vi "Initialize Components.vi"(7 "Components":refnum<class "Component.lvclass">[](array[class]), 8 "error in (no error)":errorcluster, 10 "Plugin Configuration":refnum<class "Plugin Configuration.lvclass">, 11 "Plugin Thread in":refnum<class "Plugin Thread.lvclass">) -> (0 "error out":errorcluster, 3 "Plugin Thread out":refnum<class "Plugin Thread.lvclass">)   [LabVIEW 2019, in "DSF Core.lvlib" / "Plugin Thread.lvclass"]
uses:
  Plugin Thread.lvclass
  Component/Component.lvclass
  Configuration/Core/Plugin/Plugin Configuration.lvclass
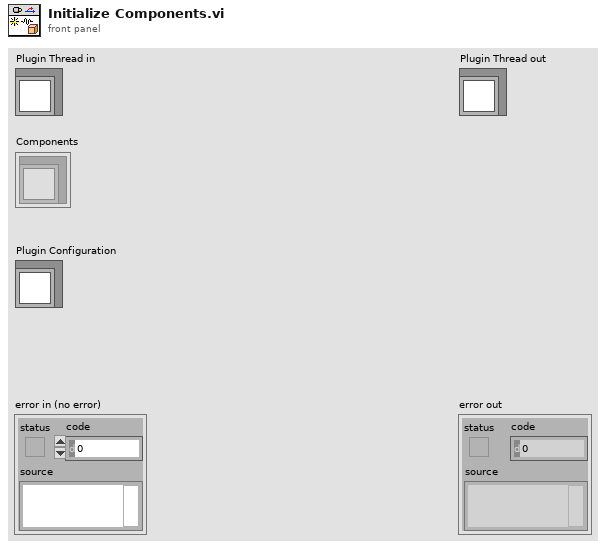
[diagram p1: front panel]
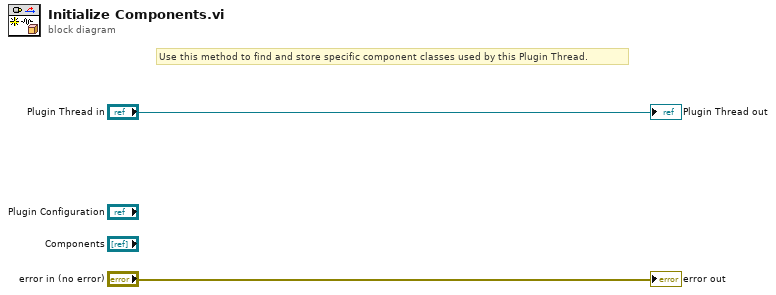
[diagram p0: block diagram]
diagram:
  # "Use this method to find and store specific component classes used by this Plugin Thread."
  "error out" <- "error in (no error)"
  "Plugin Thread out" <- "Plugin Thread in"
